vi "line_follower.vi"() -> ()   [LabVIEW 2017]
panel:
  out "Right":bool
  out "Left":bool
  out "Straight":bool
  in  "Output From Sensor 2":dbl
  in  "Output From sensor 1":dbl
  out "?":string
  out "Voltage 2":dbl
  out "Voltage 1":dbl
  in  "stop":bool
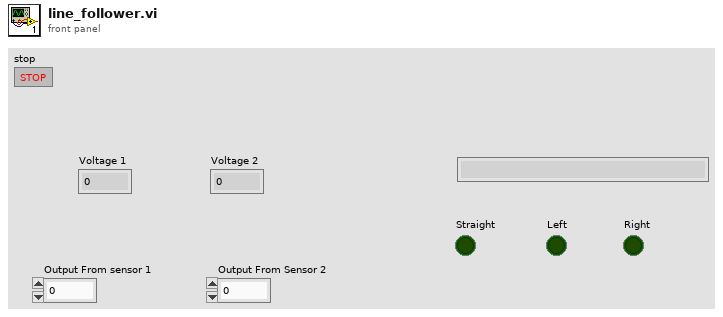
[diagram p1: front panel]
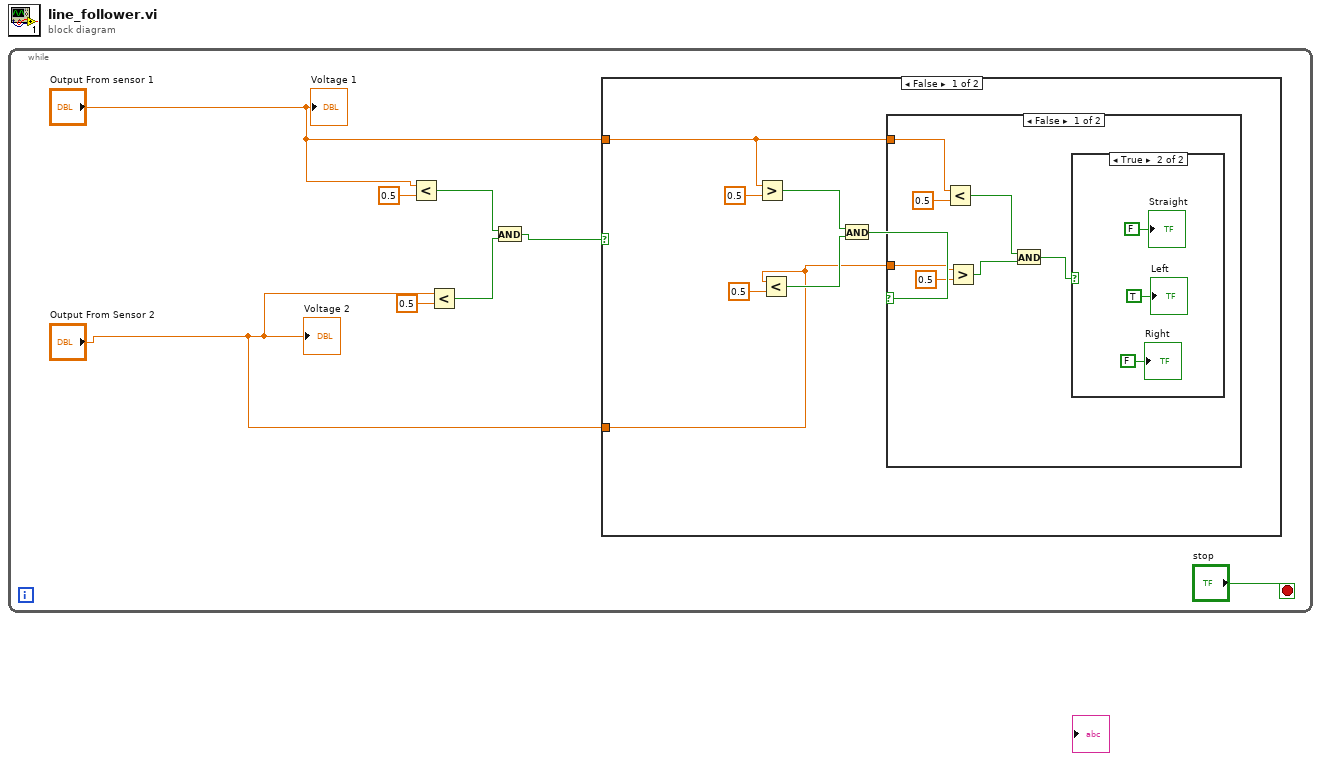
[diagram p0: block diagram]
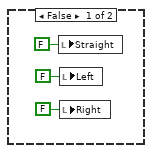
[diagram p2: hidden frame]
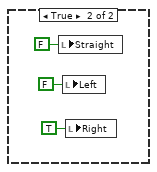
[diagram p3: hidden frame]
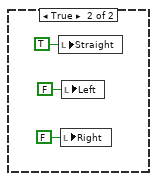
[diagram p4: hidden frame]
diagram:
  n1 = while {
    stop <- "stop" stop-if-true
    n2 = Less?(x="Output From sensor 1", y=0.5) -> (x < y?=w5:bool)
    n3 = Less?(x="Output From Sensor 2", y=0.5) -> (x < y?=w4:bool)
    n4 = And(x=w5, y=w4) -> (x .and. y?=w3:bool)
    n5 = case shown="False" w3 {
      tunnel: "Output From sensor 1" -> [w10 _]
      tunnel: "Output From Sensor 2" -> [w9 _]
      frame False {
        n6 = Greater?(x=w10, y=0.5) -> (0:w13:bool)
        n7 = Less?(x=w9, y=0.5) -> (x < y?=w12:bool)
        n8 = And(x=w13, y=w12) -> (x .and. y?=w11:bool)
        n9 = case shown="False" w11 {
          tunnel: w10 -> [w17 _]
          tunnel: w9 -> [w16 _]
          frame False {
            n10 = Less?(x=w17, y=0.5) -> (x < y?=w21:bool)
            n11 = Greater?(x=w16, y=0.5) -> (0:w20:bool)
            n12 = And(x=w21, y=w20) -> (x .and. y?=w22:bool)
            n13 = case shown="True" w22 {
              frame False {
                n14 = local write "Straight"(FALSE ("Straight")) -> ()
                n15 = local write "Left"(FALSE ("Left")) -> ()
                n16 = local write "Right"(FALSE ("Right")) -> ()
              }
              frame True {
                "Straight" <- FALSE ("Straight")
                "Left" <- TRUE ("Left")
                "Right" <- FALSE ("Right")
              }
            }
          }
          frame True {
            n17 = local write "Straight"(FALSE ("Straight")) -> ()
            n18 = local write "Left"(FALSE ("Left")) -> ()
            n19 = local write "Right"(TRUE ("Right")) -> ()
          }
        }
      }
      frame True {
        n20 = local write "Straight"(TRUE ("Straight")) -> ()
        n21 = local write "Right"(FALSE ("Right")) -> ()
        n22 = local write "Left"(FALSE ("Left")) -> ()
      }
    }
    "Voltage 1" <- "Output From sensor 1"
    "Voltage 2" <- "Output From Sensor 2"
  }
